vi "WriteSF_one.vi"(2 "payload":u8[](array[numeric]), 3 "destination ID":u16, 4 "connection ID in":refnum<k5>) -> (0 "error out":errorcluster, 1 "connection ID out":refnum<k5>)   [LabVIEW 2011]
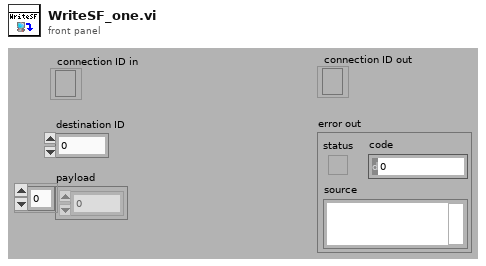
[diagram p1: front panel]
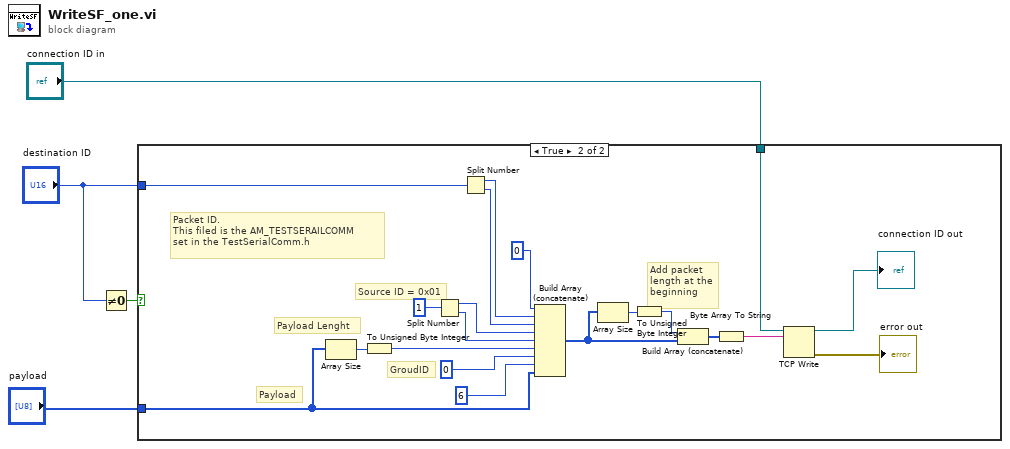
[diagram p0: block diagram]
diagram:
  n1 = Not Equal To 0?(x="destination ID") -> (x != 0?=w4:bool)
  n2 = case shown="True" w4 {
    tunnel: "destination ID" -> [_ w9]
    tunnel: "payload" -> [_ w7]
    tunnel: "connection ID in" -> [_ w6]
    frame False {
    }
    frame True {
      # "Add packet\nlength at the\nbeginning"
      # "Payload"
      # "Packet ID.\nThis filed is the AM_TESTSERAILCOMM \nset in the TestSerialComm.h"
      # "GroudID"
      # "Payload Lenght"
      # "Source ID = 0x01"
      n3 = Array Size(array=w7) -> (size(s)=w19:i32)
      n4 = To Unsigned Byte Integer(number=w19) -> (unsigned 8bit integer=w18:u8)
      n5 = Split Number(x=u16 1 ("Actuator ID\nBlue")) -> (hi(x)=w12:u8, lo(x)=w11:u8)
      n6 = Split Number(x=w9) -> (hi(x)=w21:u8, lo(x)=w20:u8)
      n7 = Build Array (concatenate)(u8 0, w21, w20, w12, w11, w18, u8 0, u8 6, w7) -> (w16:u8[])
      n8 = Array Size(array=w16) -> (size(s)=w15:i32)
      n9 = To Unsigned Byte Integer(number=w15) -> (unsigned 8bit integer=w14:u8)
      n10 = Build Array (concatenate)(w14, w16) -> (w13:u8[])
      n11 = Byte Array To String(unsigned byte array=w13) -> (string=w17:string)
      n12 = TCP Write(connection ID=w6, data in=w17) -> (connection ID out=→"connection ID out":refnum<k5>, error out=→"error out":errorcluster)  [unwired: 2 in, 1 out]
    }
  }
